vi "Init Data.vi"() -> (3 "Data Out":T1 {"LogStartTime" format="%<%x %.3X>T"})   [LabVIEW 2023]
uses:
  controls/UI Data.ctl
  <vilib>/NI/Modbus Library/API/Master/Modbus Master.lvclass
  LibreVNA/LibreVNA.lvclass
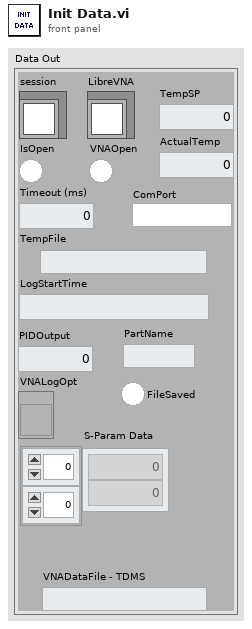
[diagram p1: front panel]
types:
  T1 = typedef "UI Data.ctl" = cluster{"session":refnum<class "Modbus Master.lvclass">, "IsOpen":bool, "Timeout (ms)":i32, "TempFile":path, "LogStartTime":timestamp, "LibreVNA":refnum<class "LibreVNA.lvclass">, "VNAOpen":bool, "TempSP":dbl, "ActualTemp":dbl, "FileSaved":bool, "PIDOutput":dbl, "VNALogOpt":refnum<vi>, "PartName":string, "ComPort":refnum<visa-resource-name>, "S-Param Data":dbl[][], "VNADataFile - TDMS":path}
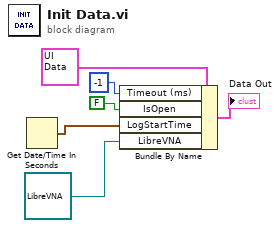
[diagram p0: block diagram]
diagram:
  n1 = Get Date/Time In Seconds() -> (seconds since 1Jan1904=w2:timestamp)
  n2 = Bundle By Name(cluster=T1 {"session"=refnum, "IsOpen"=FALSE, "Timeout (ms)"=0, "TempFile"=path "", "LogStartTime"=timestamp(0 s since 1904-01-01), "LibreVNA"=refnum, "VNAOpen"=FALSE, "TempSP"=0.0, "ActualTemp"=0.0, "FileSaved"=FALSE, "PIDOutput"=0.0, "VNALogOpt"=refnum, "PartName"="", "ComPort"="", "S-Param Data"=[], "VNADataFile - TDMS"=path ""} ("Data Cluster"), "Timeout (ms)"=-1, "IsOpen"=FALSE, "LogStartTime"=w2, "LibreVNA"=refnum<class "LibreVNA.lvclass"> refnum) -> (→"Data Out":T1)
